vi "asset.create.vi"(8 "error in":errorcluster, 9 "description":string, 10 "name":string, 11 "Client in":refnum<class "Client.lvclass">) -> (0 "error out":errorcluster, 2 "Asset":refnum<class "Asset.lvclass">, 3 "Client out":refnum<class "Client.lvclass">)   [LabVIEW 2020, in "Client.lvclass"]
doc: "Creates a new asset in Nominal with the given name and optional description, and returns a handle to it."
uses:
  Client.lvclass
  Asset/Asset.lvclass
  Client.lvclass/Client.ctl
  Asset/Asset.lvclass/Asset.ctl
  client.lvlib
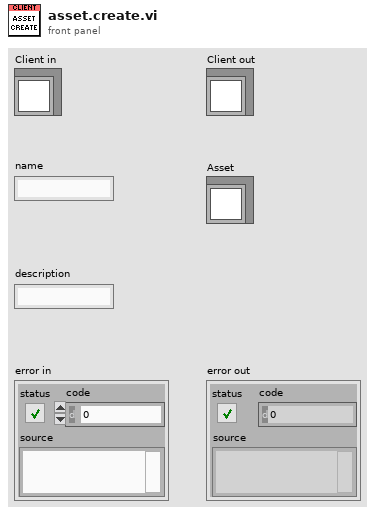
[diagram p1: front panel]
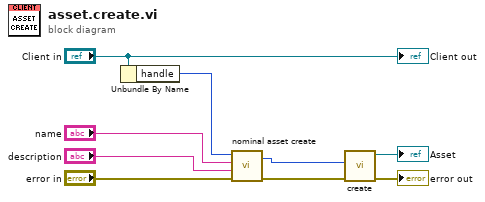
[diagram p0: block diagram]
diagram:
  n1 = Unbundle By Name("Client in") -> ("handle"=w8:i32)
  n2 = call "nominal asset create.vi"("error in (no error)"="error in", "description"="description", "name"="name", "client"=w8) -> ("error out"=w2:errorcluster, "out_asset out"=w3:i32)  [unwired: 5 in, 1 out]
  n3 = call "create.vi"("error in (no error)"=w2, "handle"=w3) -> ("error out"=→"error out":errorcluster, "Asset out"=→"Asset":refnum<class "Asset.lvclass">)  [unwired: 8 in]
  "Client out" <- "Client in"
